vi "New Test Suite.vi"() -> ()   [LabVIEW 2011]
uses:
  Libraries/VITesterUtilities.lvlib
panel:
  out "error out":errorcluster
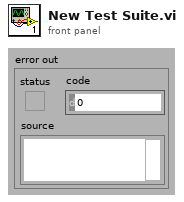
[diagram p1: front panel]
types:
  T1 = typedef "Menu Launch Info - Cluster__jki_lib_application_control -- VI Tester.ctl" = cluster{"Application":refnum<vi>, "Selected Project Items":T2[]}
  T2 = typedef "Project Item Info - Cluster__jki_lib_application_control -- VI Tester.ctl" = cluster{"Type":string, "Name":string, "Path":path}
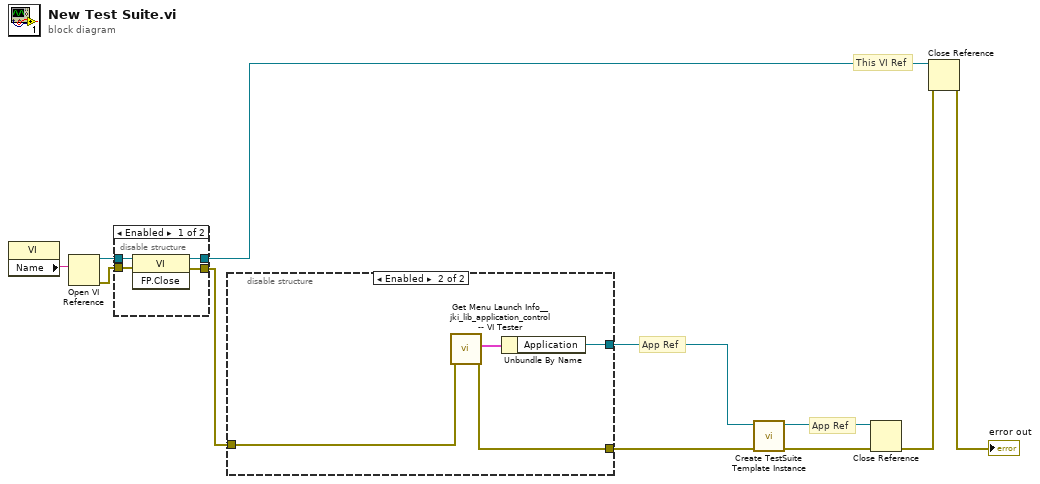
[diagram p0: block diagram]
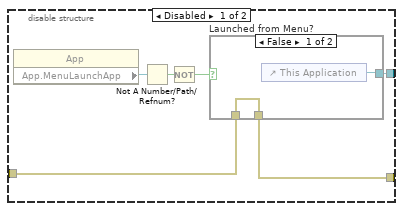
[diagram p2: hidden frame]
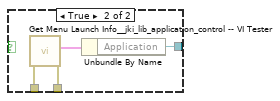
[diagram p3: hidden frame]
diagram:
  # "This VI Ref"
  # "App Ref"
  # "App Ref"
  n1 = property class="VI"() -> ("Name"=w11:string)  [unwired: 2 in, 2 out]
  n2 = Open VI Reference(vi path=w11) -> (vi reference=w10:refnum<vi>, error out=w8:errorcluster)  [unwired: 5 in]
  n3 = disable-structure shown="Enabled" {
    disable-tunnel: [w15 w16] -> w5
    disable-tunnel: w10 -> [w14 w17]
    disable-tunnel: [w13 w17] -> w9
    disable-tunnel: w8 -> [w12 w16]
    frame Enabled {
      n4 = invoke class="VI" method="FP.Close"(reference=w14, error in=w12) -> (reference out=w13:refnum<vi>, error out=w15:errorcluster)  [unwired: 1 in, 1 out]
    }
    frame Disabled {
    }
  }
  n5 = disable-structure shown="Enabled" {
    disable-tunnel: [w20 w33] -> w4
    disable-tunnel: w5 -> [w19 w32]
    disable-tunnel: [w18 w31] -> w3
    frame Disabled {
      n6 = property class="App"() -> ("App.MenuLaunchApp"=w23:refnum<vi>)  [unwired: 2 in, 2 out]
      n7 = Not A Number/Path/Refnum?(number/path/refnum=w23) -> (NaN/Path/Refnum?=w22:bool)
      n8 = Not(x=w22) -> (.not. x?=w21:bool)
      n9 = case "Launched from Menu?" shown="False" w21 {
        tunnel: [w25 w28] -> w20
        tunnel: [w24 w27] -> w18
        tunnel: w19 -> [w24 w26]
        frame False {
          n10 = control-ref of="This Application"() -> (w25:refnum<vi>)
        }
        frame True {
          n11 = call "Get Menu Launch Info__jki_lib_application_control -- VI Tester.vi"("error in (no error)"=w26) -> ("error out"=w27:errorcluster, "Menu Launch info"=w29:T1)  [unwired: 9 in]
          n12 = Unbundle By Name(w29) -> ("Application"=w28:refnum<vi>)
        }
      }
    }
    frame Enabled {
      n13 = call "Get Menu Launch Info__jki_lib_application_control -- VI Tester.vi"("error in (no error)"=w32) -> ("error out"=w31:errorcluster, "Menu Launch info"=w30:T1)  [unwired: 9 in]
      n14 = Unbundle By Name(w30) -> ("Application"=w33:refnum<vi>)
    }
  }
  n15 = call "Create TestSuite Template Instance.vi"("error in"=w3, "Application Ref (This Application)"=w4) -> ("error out"=w2:errorcluster, "Application Ref"=w1:refnum<vi>)  [unwired: 8 in]
  n16 = Close Reference(reference=w1, error in (no error)=w2) -> (error out=w7:errorcluster)
  n17 = Close Reference(reference=w9, error in (no error)=w7) -> (error out=→"error out":errorcluster)
